vi "Data Type.vi"() -> ()   [LabVIEW 2020]
panel:
  out "I 33":i32
  out "U 33":u32
  out "I 17":i16
  out "U 17":u16
  in  "I 32":i32
  in  "U 32":u32
  in  "I 16":i16
  in  "U 16":u16
  out "I8 2":i8
  out "U8":u8
  in  "I8":i8
  in  "U8":u8
  # "Data Type"
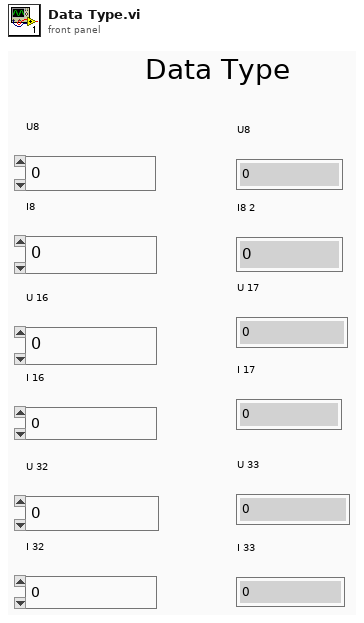
[diagram p1: front panel]
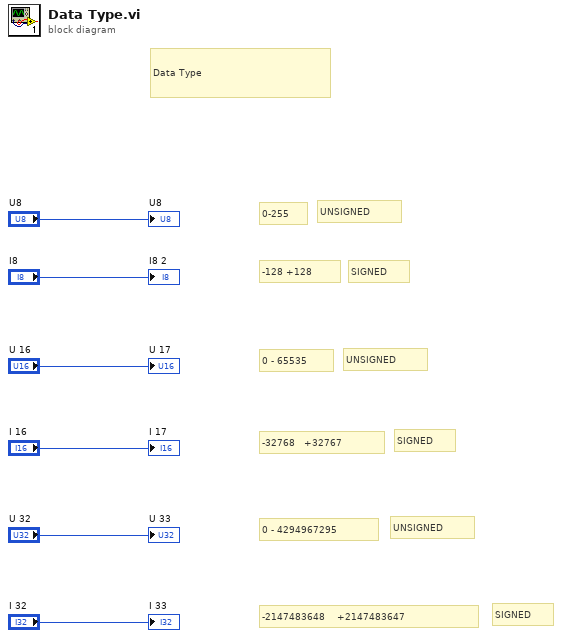
[diagram p0: block diagram]
diagram:
  # "Data Type"
  # "UNSIGNED"
  # "UNSIGNED"
  # "SIGNED"
  # "SIGNED"
  # "SIGNED"
  # "UNSIGNED"
  # "-2147483648    +2147483647"
  # "0 - 4294967295"
  # "-32768   +32767"
  # "0 - 65535"
  # "-128 +128"
  # "0-255"
  "U8" <- "U8"
  "I8 2" <- "I8"
  "U 17" <- "U 16"
  "I 17" <- "I 16"
  "U 33" <- "U 32"
  "I 33" <- "I 32"
